vi "Edit(Channel).vi"(10 "TaskConfig":refnum<data-value>, 11 "Tag":string) -> ()   [LabVIEW 2025, in "DAQ_Module.lvlib" / "DAQ_Module.lvclass"]
uses:
  DAQ_Module.lvclass
  DAQ_Config.ctl
  DAQ_Task_Config.ctl
  DAQ_HW_Type.ctl
  DAQ_Task_Type.ctl
  DAQ_SampleRateConfig.ctl
  DAQ_AI_Task_Config.ctl
  DAQ_Linear_Task_Config.ctl
  DAQ_Angular_Task_Config.ctl
  <vilib>/addons/_JKI Toolkits/State Machine/_JKI_lib_State_Machine.llb/Select State(s)_err__jki_lib_state_machine.vi
  <vilib>/addons/_JKI Toolkits/State Machine/_JKI_lib_State_Machine.llb/Periodic Trigger__ogtk__JKI-SM__jki_lib_state_machine.vi
panel:
  in  "Cancel":bool
  in  "OK":bool
  in  "Tab Control":enum32{"AI", "Linear", "Angular", "AO"}(tab)
  in  "AI_Config":T1={"AI"={"MaxValue"=1.0, "MinValue"=0.0, "InputTerminalConfiguration"=-1}, "Scale"={"Offset"=0.0, "Gain"=1.0, "Unit"=""}, "Calibrate"={"K"=0.0, "B"=1.0}} {"AI"."InputTerminalConfiguration" items=["default"=-1, "RSE"=10083, "NRSE"=10078, "Differential"=10106, "Pseudodifferential"=12529]}
  in  "LinearConfig":T2={"decoding type"=10092, "units"=10219, "distance per pulse"=0.001, "initial position"=0.0, "z index enable"=FALSE, "z index value"=0.0, "z index phase"=10040, "CI_Encoder_A_InputTerm"="", "CI_Encoder_B_InputTerm"="", "CI_Encoder_Z_InputTerm"=""} {"units" items=["Meters"=10219, "Inches"=10379, "Ticks"=10304, "From Custom Scale"=10065]; "decoding type" items=["X1"=10090, "X2"=10091, "X4"=10092, "Two Pulse Counting"=10313]; "z index phase" items=["A High B High"=10040, "A High B Low"=10041, "A Low B High"=10042, "A Low B Low"=10043]}
  in  "AngularConfig":T3={"decoding type"=10092, "units"=10146, "pulses per revolution"=24, "initial angle"=0.0, "z index enable"=FALSE, "z index value"=0.0, "z index phase"=10040, "CI_Encoder_A_InputTerm"="", "CI_Encoder_B_InputTerm"="", "CI_Encoder_Z_InputTerm"=""} {"units" items=["Degrees"=10146, "Radians"=10273, "Ticks"=10304, "From Custom Scale"=10065]; "decoding type" items=["X1"=10090, "X2"=10091, "X4"=10092, "Two Pulse Counting"=10313]; "z index phase" items=["A High B High"=10040, "A High B Low"=10041, "A Low B High"=10042, "A Low B Low"=10043]}
  in  "Name":string
  in  "Channel":string
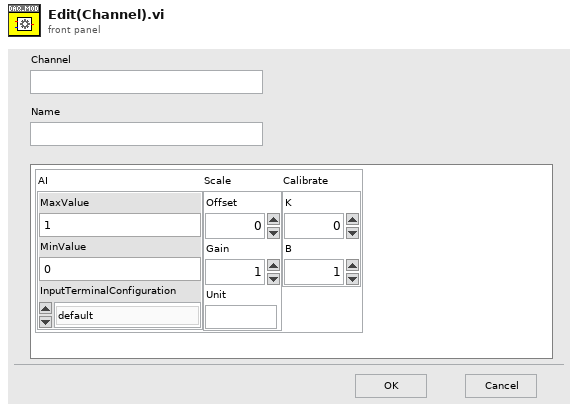
[diagram p1: front panel]
types:
  T1 = typedef "DAQ_Module.lvlib/DAQ_Module.lvclass/DAQ_AI_Task_Config.ctl" = cluster{"AI":cluster{"MaxValue":dbl, "MinValue":dbl, "InputTerminalConfiguration":i32}, "Scale":cluster{"Offset":dbl, "Gain":dbl, "Unit":string}, "Calibrate":cluster{"K":dbl, "B":dbl}}
  T2 = typedef "DAQ_Module.lvlib/DAQ_Module.lvclass/DAQ_Linear_Task_Config.ctl" = cluster{"decoding type":i32, "units":i32, "distance per pulse":dbl, "initial position":dbl, "z index enable":bool, "z index value":dbl, "z index phase":i32, "CI_Encoder_A_InputTerm":string, "CI_Encoder_B_InputTerm":string, "CI_Encoder_Z_InputTerm":string}
  T3 = typedef "DAQ_Module.lvlib/DAQ_Module.lvclass/DAQ_Angular_Task_Config.ctl" = cluster{"decoding type":i32, "units":i32, "pulses per revolution":u32, "initial angle":dbl, "z index enable":bool, "z index value":dbl, "z index phase":i32, "CI_Encoder_A_InputTerm":string, "CI_Encoder_B_InputTerm":string, "CI_Encoder_Z_InputTerm":string}
  T4 = enum32{"Invalid", "Standard", "Closed", "Hidden", "Minimized", "Maximized"}
  T5 = enum32{"invalid app kind", "Development System", "Run Time System", "Student Edition", "Embedded LabVIEW", "Evaluation", "Custom"}
  T6 = cluster{"Core":cluster{"Current VI Reference":refnum<vi>, "Close Panel on Exit?":bool}, "TaskConfig":refnum<data-value>, "Tag":string, "AI_Config":refnum<vi>, "AngularConfig":refnum<vi>, "LinearConfig":refnum<vi>, "Tab Control":refnum<vi>, "Channel":refnum<vi>, "Name":refnum<vi>}
  T7 = cluster{"Current VI Reference":refnum<vi>, "Close Panel on Exit?":bool}
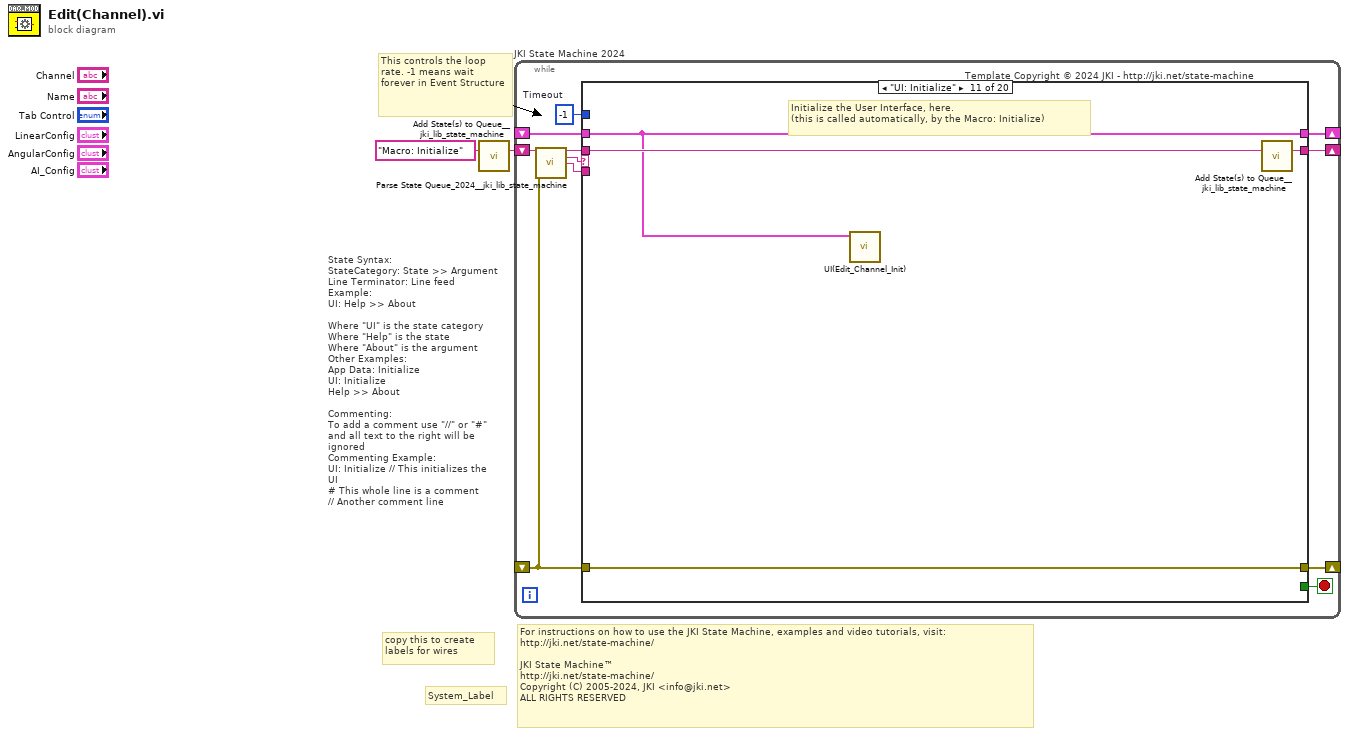
[diagram p0: block diagram]
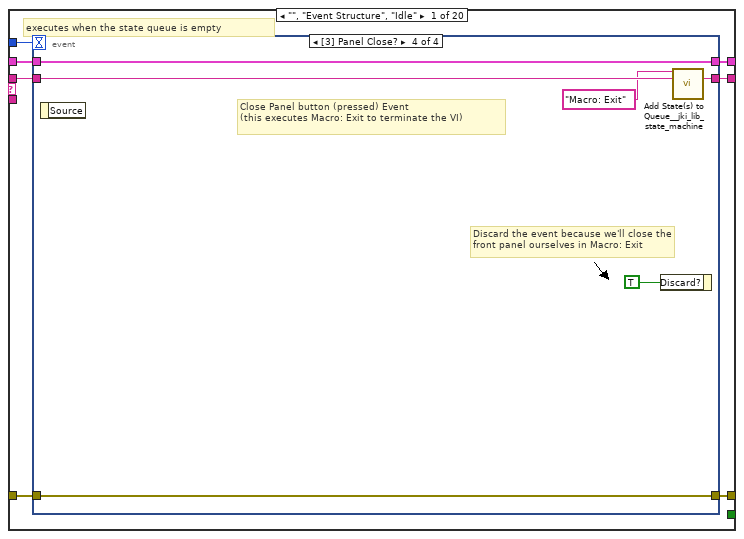
[diagram p2: hidden frame]
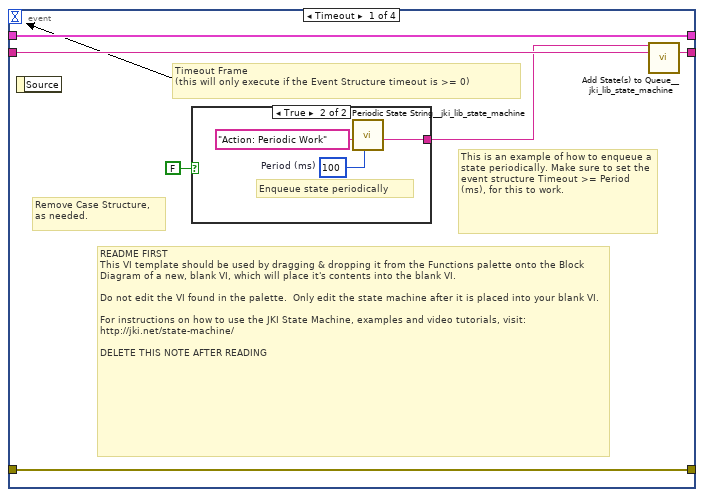
[diagram p3: hidden frame]
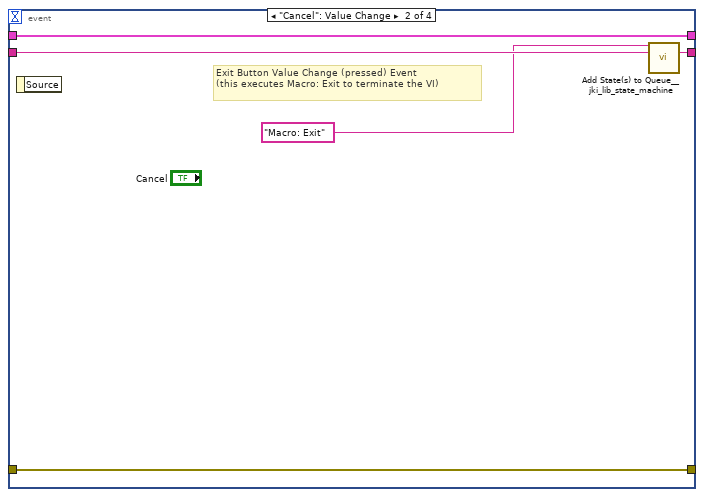
[diagram p5: hidden frame]
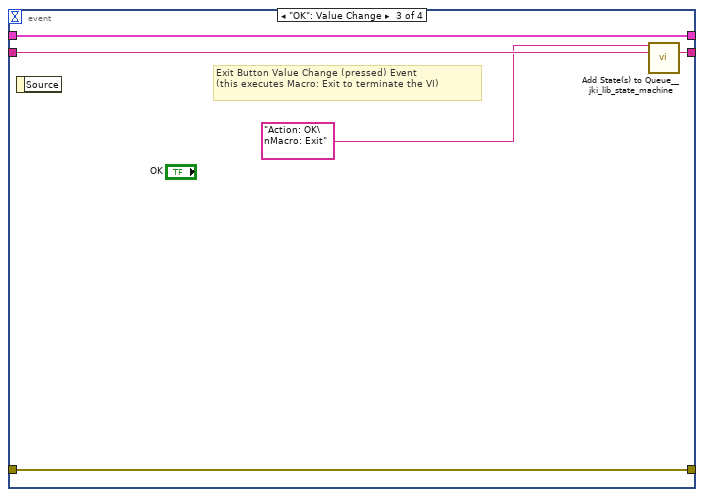
[diagram p6: hidden frame]
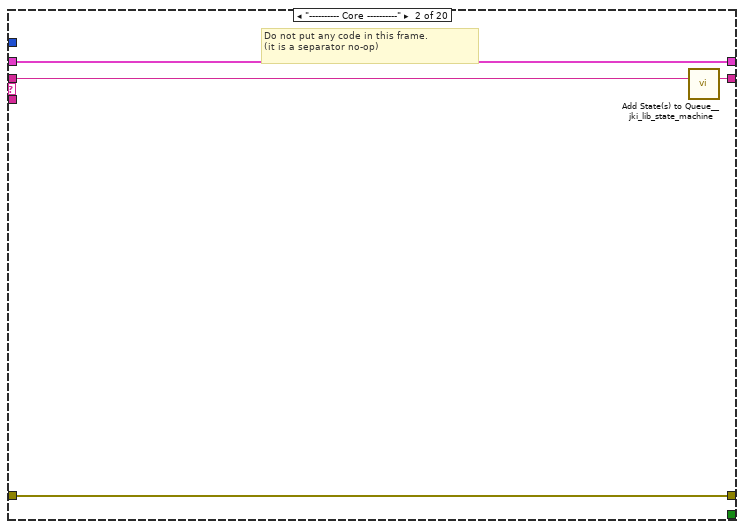
[diagram p7: hidden frame]
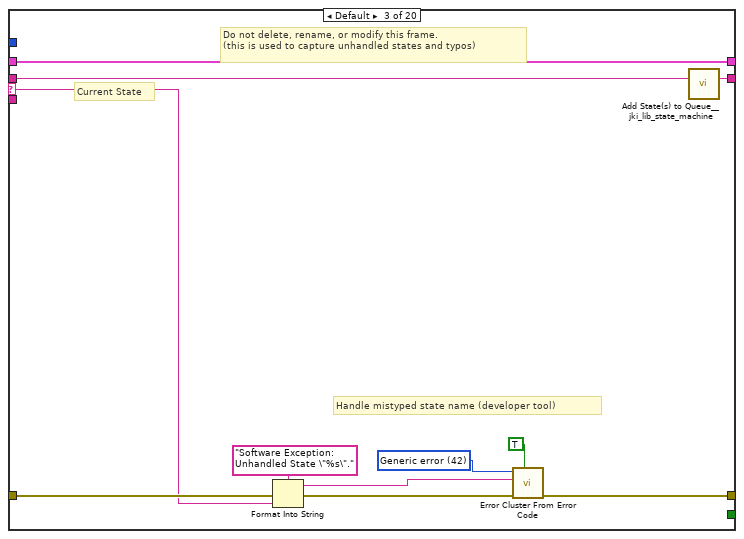
[diagram p8: hidden frame]
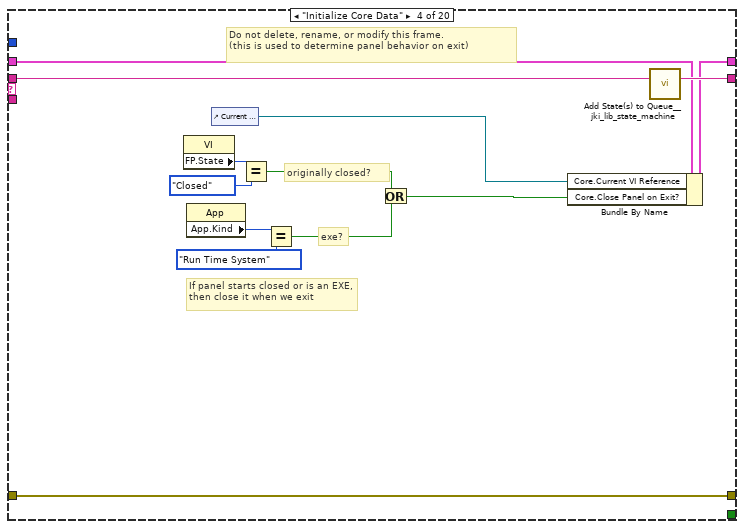
[diagram p9: hidden frame]
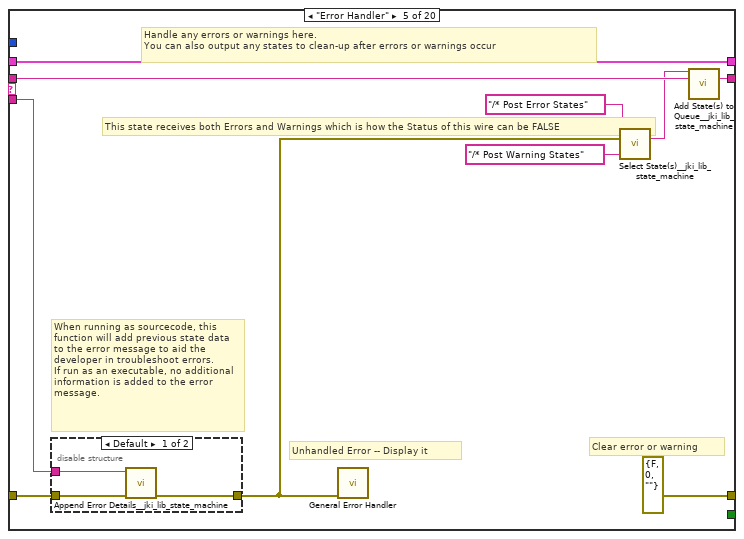
[diagram p10: hidden frame]
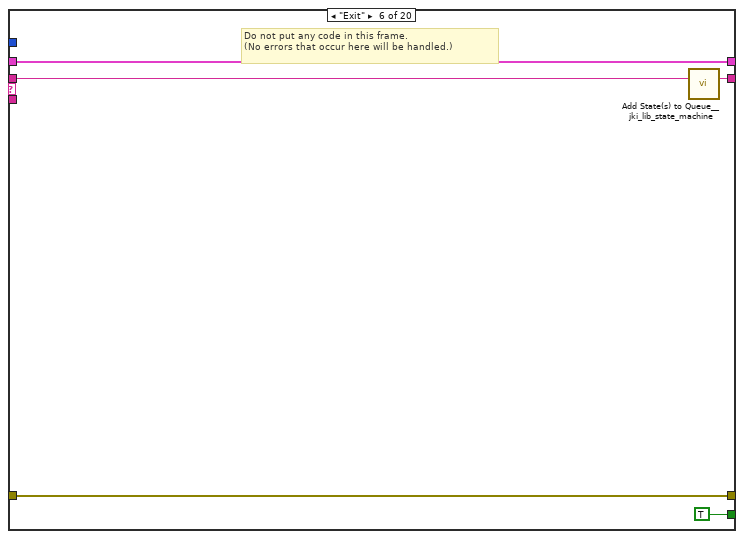
[diagram p12: hidden frame]
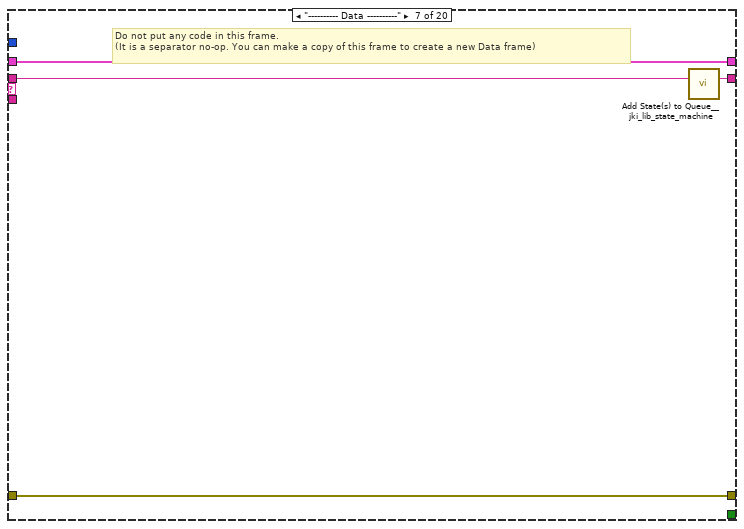
[diagram p13: hidden frame]
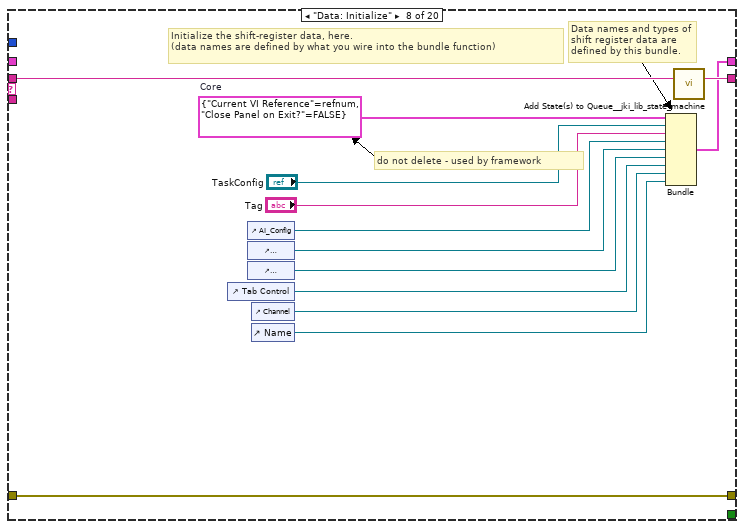
[diagram p14: hidden frame]
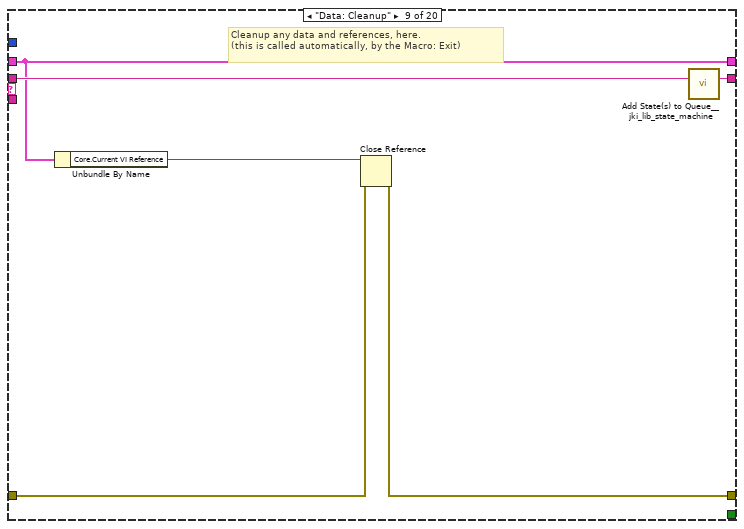
[diagram p15: hidden frame]
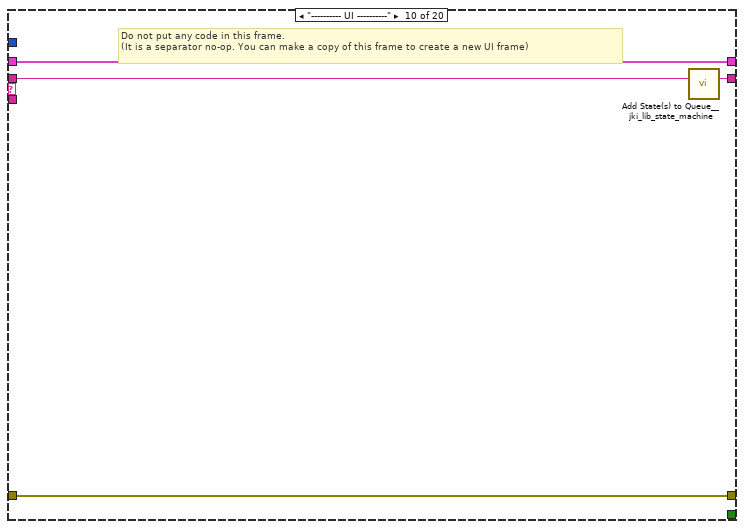
[diagram p16: hidden frame]
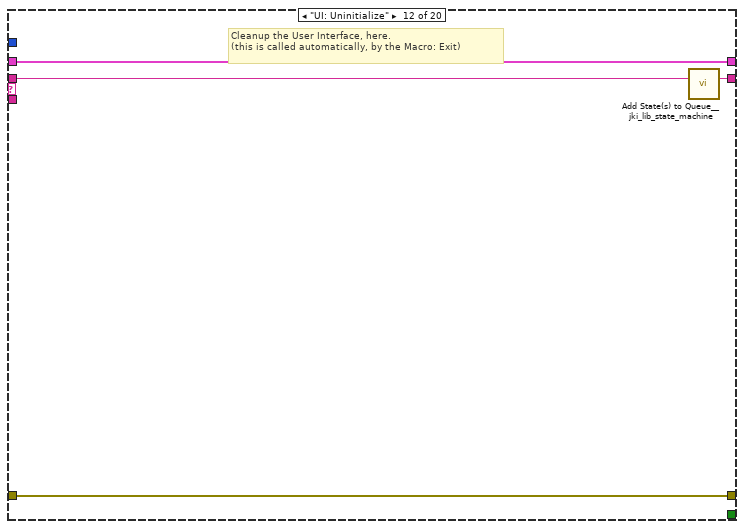
[diagram p17: hidden frame]
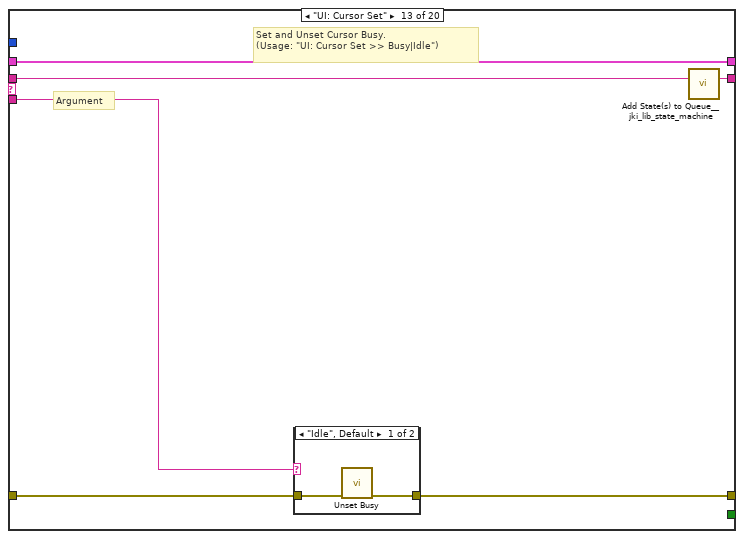
[diagram p18: hidden frame]
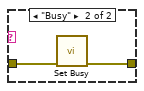
[diagram p19: hidden frame]
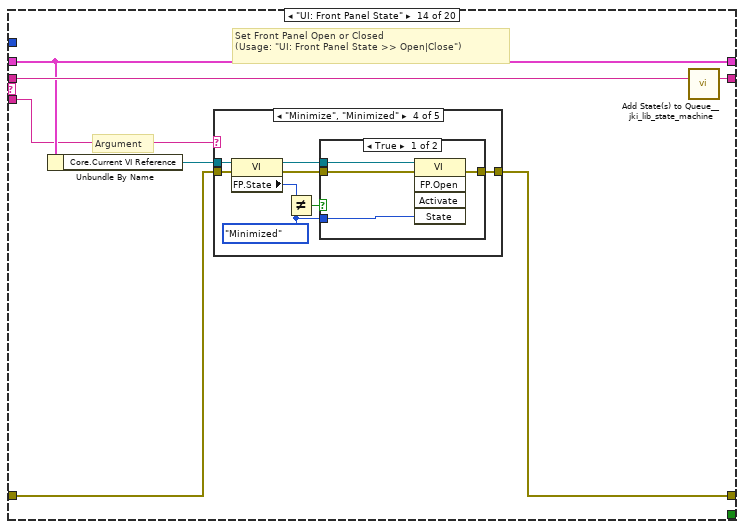
[diagram p20: hidden frame]
diagram:
  # "For instructions on how to use the JKI State Machine, examples and video tutorials, visit:\nhttp://jki.net/state-machine/\n\nJKI State Machine™\nhttp://jki.net/state-machine/\nCopyright (C) 2005-2024, JKI <info@jki.net>\nALL RIGHTS RESERVED"
  # "State Syntax:\nStateCategory: State >> Argument\nLine Terminator: Line feed\nExample:\nUI: Help >> About\n\nWhere \"UI\" is the state category\nWhere \"Help\" is the state\nWhere \"About\" is the argument\nOther Examples:\nApp Data: Initialize\nUI: Initialize\nHelp >> About\n\nCommenting:\nTo add a comment use \"//\" or \"#\" and all text to the right will be ignored\nCommenting Example:\nUI: Initialize // This initializes the UI\n# This whole line is a comment\n// Another comment line"
  # "copy this to create labels for wires"
  # "This controls the loop rate. -1 means wait forever in Event Structure"
  # "System_Label"
  n1 = call <vilib>:"Add State(s) to Queue__jki_lib_state_machine.vi"("State(s) in (\"\")"="Macro: Initialize") -> ("States Out"=w2:string)  [unwired: 14 in]
  n2 = while "JKI State Machine 2024" {
    shift-right: [w6] -> _
    shift-left: _ -> [w5]
    shift-right: [w9] -> _
    shift-left: _ -> [w3]
    shift-right: [w8] -> _
    shift-left: w2 -> [w10]
    stop <- w7 stop-if-true
    w4 = -1  # Timeout
    # "Template Copyright © 2024 JKI - http://jki.net/state-machine"
    n3 = call <vilib>:"Parse State Queue_2024__jki_lib_state_machine.vi"("State Queue"=w10, "Error In (no error)"=w3) -> ("Remaining States"=w12:string, "Current State"=w13:string, "Arguments"=w11:string)  [unwired: 11 in]
    n4 = case shown="\"UI: Initialize\"" w13 {
      selector: w13 -> [_ _ w50 _ _ _ _ _ _ _ _ _ _ _ _ _ _ _ _ _]
      tunnel: w12 -> [w20 w49 w54 w73 w83 w92 w96 w109 w115 w119 w123 w127 w133 w144 w213 w218 w227 w231 w235 w239]
      tunnel: w11 -> [_ _ _ _ w78 _ _ _ _ _ _ _ w128 w138 _ _ _ _ _ _]
      tunnel: w5 -> [w18 w46 w52 w66 w80 w90 w93 _ w110 w116 w120 w125 w131 w140 w210 w215 w225 w228 w232 w236]
      tunnel: [w17 w47 w56 w70 errorcluster {"status"=FALSE, "code"=0, "source"=""} ("error out") w89 w94 w106 w111 w117 w121 w124 w129 w141 w211 w216 w222 w229 w233 w237] -> w9
      tunnel: w3 -> [w14 w47 w55 w70 w79 w89 w94 w106 w112 w117 w121 w124 w130 w142 w211 w216 w222 w229 w233 w237]
      tunnel: [w19 w48 w53 w72 w82 w91 w95 w108 w114 w118 w122 w126 w132 w143 w212 w217 w226 w230 w234 w238] -> w8
      tunnel: [_ _ _ _ _ TRUE _ _ _ _ _ _ _ _ _ _ _ _ _ _] -> w7
      tunnel: [w16 w46 w52 w71 w80 w90 w93 w107 w110 w116 w120 w125 w131 w140 w210 w215 w225 w228 w232 w236] -> w6
      tunnel: w4 -> [w15 _ _ _ _ _ _ _ _ _ _ _ _ _ _ _ _ _ _ _]
      frame "", "Event Structure", "Idle" {
        # "executes when the state queue is empty"
        n5 = event shown="[3] Panel Close?" {
          selector: _ -> [_ _ _ _]
          dyn-events: _ -> [_ _ _ _]
          timeout: w15 -> [_ _ _ _]
          tunnel: w20 -> [w26 w34 w39 w45]
          tunnel: [w25 w33 w38 w44] -> w19
          tunnel: w18 -> [w23 w31 w36 w42]
          tunnel: [w24 w32 w37 w43] -> w17
          tunnel: w14 -> [w24 w32 w37 w43]
          tunnel: [w23 w31 w36 w42] -> w16
          event Timeout {
            # "Remove Case Structure, as needed."
            # "This is an example of how to enqueue a state periodically. Make sure to set the event structure Timeout >= Period (ms), for this to work."
            # "README FIRST\nThis VI template should be used by dragging & dropping it from the Functions palette onto the Block Diagram of a new, blank VI, which will place it's contents into the blank VI.\n\nDo not edit the VI found in the palette.  Only edit the state machine after it is placed into your blank VI.\n\nFor instructions on how to use the JKI State Machine, examples and video tutorials, visit:\nhttp://jki.net/state-machine/\n\nDELETE THIS NOTE AFTER READING"
            # "Timeout Frame\n(this will only execute if the Event Structure timeout is >= 0)"
            n6 = event-data() -> ()  [unwired: 1 in, 1 out]
            n7 = case shown="True" FALSE {
              tunnel: [_ w29] -> w22
              frame False {
              }
              frame True {
                w27 = u32 100  # Period (ms)
                # "Enqueue state periodically"
                n8 = call <vilib>:"Periodic State String__jki_lib_state_machine.vi"("Period (ms)"=w27, "State"="Action: Periodic Work") -> ("State Out"=w29:string)  [unwired: 9 in]
              }
            }
            n9 = call <vilib>:"Add State(s) to Queue__jki_lib_state_machine.vi"("State(s) in Front (\"\")"=w22, "State(s) in (\"\")"=w26) -> ("States Out"=w25:string)  [unwired: 13 in]
          }
          event "Cancel": Value Change {
            # "Exit Button Value Change (pressed) Event\n(this executes Macro: Exit to terminate the VI)"
            n10 = event-data() -> ()  [unwired: 1 in, 1 out]
            n11 = call <vilib>:"Add State(s) to Queue__jki_lib_state_machine.vi"("State(s) in Front (\"\")"="Macro: Exit", "State(s) in (\"\")"=w34) -> ("States Out"=w33:string)  [unwired: 13 in]
          }
          event "OK": Value Change {
            # "Exit Button Value Change (pressed) Event\n(this executes Macro: Exit to terminate the VI)"
            n12 = event-data() -> ()  [unwired: 1 in, 1 out]
            n13 = call <vilib>:"Add State(s) to Queue__jki_lib_state_machine.vi"("State(s) in Front (\"\")"="Action: OK\nMacro: Exit", "State(s) in (\"\")"=w39) -> ("States Out"=w38:string)  [unwired: 13 in]
          }
          event Panel Close? {
            # "Discard the event because we'll close the front panel ourselves in Macro: Exit"
            # "Close Panel button (pressed) Event\n(this executes Macro: Exit to terminate the VI)"
            n14 = event-data() -> ()  [unwired: 1 in, 1 out]
            n15 = event-data("Discard?"=TRUE) -> ()  [unwired: 1 in, 1 out]
            n16 = call <vilib>:"Add State(s) to Queue__jki_lib_state_machine.vi"("State(s) in Front (\"\")"="Macro: Exit", "State(s) in (\"\")"=w45) -> ("States Out"=w44:string)  [unwired: 13 in]
          }
        }
      }
      frame "---------- Core ----------" {
        # "Do not put any code in this frame.\n(it is a separator no-op)"
        n17 = call <vilib>:"Add State(s) to Queue__jki_lib_state_machine.vi"("State(s) in (\"\")"=w49) -> ("States Out"=w48:string)  [unwired: 14 in]
      }
      frame Default {
        w59 = 42 items=["No error", "Argument error", "Memory is full", "Out of zone", "End of file", "File already open", "Generic file I/O error", "File not found", "File permission error", "Disk is full", "Duplicate path", "Too many files open", "System feature not enabled", "Resource file not found", "Cannot add resource", "Resource not found", "Image not found", "Image memory error", "Pen does not exist", "Config type invalid", "Config token not found", "Config parse error", "Config memory error", "Bad external code format", "Bad external code offset", "External code not present", "Null window", "Destroy window error", "Null menu", "Print aborted", "Bad print record", "Print driver error", "Windows error during printing", "Memory error during printing", "Print dialog error", "Generic print error", "Invalid device refnum", "Device not found", "Device parameter error", "Device unit error", "Cannot open device", "Device call aborted", "Generic error", "Cancelled by user", "Object ID too low", "Object ID too high", "Object not in heap", "Unknown heap", "Unknown object (invalid DefProc)", "Unknown object (DefProc not in table)", "Message out of range", "Invalid (null) method", "Unknown message", "Manager call not supported", "Bad address", "Network operation in progress", "Network operation timed out", "Connection is busy", "Network attribute not supported", "Network error", "Address in use", "System out of memory", "Connection aborted", "Connection refused", "Not connected", "Already connected", "Connection closed", "Initialization error (interapplication manager)", "Bad occurrence", "Wait on unbound occurrence handler", "Occurrence queue overflow", "Datalog type conflict", "Unused", "Unrecognized type (interapplication manager)", "Memory corrupt", "Failed to make temporary DLL", "Old CIN version", "Drag socket not found", "Failed to load drop-object", "Failed to register OLE object", "Failed to release OLE object", "Format specifier type mismatch", "Unknown format specifier", "Too few format specifiers", "Too many format specifiers", "Scan failed", "Newer CIN version", "Error converting to variant", "Runtime menu error", "Password tampered", "Variant attribute not found", "Incompatible variant data type", "Event data is not available", "Event Store is not present", "Occurrence is not found", "Event Queue is not created", "Event info is not available", "Refnum passed is NULL", "Error retrieving Class GUID", "Error retrieving CoClass GUID", "Error retrieving TypeLib GUID.", "Bad built application magic bytes.", "Specific driver is different from the specific driver associated with the Logical Name.", "There is no session opened to the class driver.", "Max Error", "MAX - Error with config objects", "MAX - Error loading configuration", "MAX - Group not supported"]
        # "Current State"
        # "Do not delete, rename, or modify this frame.\n(this is used to capture unhandled states and typos)"
        # "Handle mistyped state name (developer tool)"
        n18 = Format Into String(format string="Software Exception: Unhandled State \"%s\"." ("message"), error in=w55, w50) -> (resulting string=w58:string, error out=w57:errorcluster)  [unwired: 1 in]
        n19 = call <vilib>:"Error Cluster From Error Code.vi"("show call chain? (False)"=TRUE, "error in (no error)"=w57, "error message (\"\")"=w58, "error code (0)"=w59) -> ("error out"=w56:errorcluster)  [unwired: 5 in]
        n20 = call <vilib>:"Add State(s) to Queue__jki_lib_state_machine.vi"("State(s) in (\"\")"=w54) -> ("States Out"=w53:string)  [unwired: 14 in]
      }
      frame "Initialize Core Data" {
        # "Do not delete, rename, or modify this frame.\n(this is used to determine panel behavior on exit)"
        # "originally closed?"
        # "exe?"
        # "If panel starts closed or is an EXE, then close it when we exit"
        n21 = property class="VI"() -> ("FP.State"=w63:T4)  [unwired: 2 in, 2 out]
        n22 = property class="App"() -> ("App.Kind"=w69:T5)  [unwired: 2 in, 2 out]
        n23 = control-ref of="Current VI Reference"() -> (w64:refnum<vi>)
        n24 = Equal?(x=w63, y=T4."Closed" ("Front Panel Window:State")) -> (x = y?=w61:bool)
        n25 = Equal?(x=w69, y=T5."Run Time System" ("Application:Kind")) -> (x = y?=w67:bool)
        n26 = Or(x=w61, y=w67) -> (x .or. y?=w65:bool)
        n27 = Bundle By Name(cluster=w66, "Core.Current VI Reference"=w64, "Core.Close Panel on Exit?"=w65) -> (w71:T6)
        n28 = call <vilib>:"Add State(s) to Queue__jki_lib_state_machine.vi"("State(s) in (\"\")"=w73) -> ("States Out"=w72:string)  [unwired: 14 in]
      }
      frame "Error Handler" {
        # "When running as sourcecode, this function will add previous state data to the error message to aid the developer in troubleshoot errors.\nIf run as an executable, no additional information is added to the error message."
        # "This state receives both Errors and Warnings which is how the Status of this wire can be FALSE"
        # "Unhandled Error -- Display it"
        # "Handle any errors or warnings here.\nYou can also output any states to clean-up after errors or warnings occur"
        # "Clear error or warning"
        n29 = disable-structure shown="Default" {
          disable-tunnel: w79 -> [w86 w87]
          disable-tunnel: w78 -> [w85 _]
          disable-tunnel: [w84 w87] -> w77
          frame condition #0 (active) {
            n30 = call <vilib>:"Append Error Details__jki_lib_state_machine.vi"("error in (no error)"=w86, "Previous State and Argument(s)"=w85) -> ("error out"=w84:errorcluster)  [unwired: 9 in]
          }
          frame condition #1 {
          }
        }
        n31 = call <vilib>:"General Error Handler.vi"("error in (no error)"=w77) -> ()  [unwired: 10 in, 5 out]
        n32 = call-poly <vilib>:"Select State(s)__jki_lib_state_machine.vi"("State(s) if True (\"\")"="/* Post Error States", "Select"=w77, "State(s) if False (\"\")"="/* Post Warning States") -> ("States Out"=w75:string)  [unwired: 12 in]
        n33 = call <vilib>:"Add State(s) to Queue__jki_lib_state_machine.vi"("State(s) in Front (\"\")"=w75, "State(s) in (\"\")"=w83) -> ("States Out"=w82:string)  [unwired: 13 in]
      }
      frame "Exit" {
        # "Do not put any code in this frame.\n(No errors that occur here will be handled.)"
        n34 = call <vilib>:"Add State(s) to Queue__jki_lib_state_machine.vi"("State(s) in (\"\")"=w92) -> ("States Out"=w91:string)  [unwired: 14 in]
      }
      frame "---------- Data ----------" {
        # "Do not put any code in this frame.\n(It is a separator no-op. You can make a copy of this frame to create a new Data frame)"
        n35 = call <vilib>:"Add State(s) to Queue__jki_lib_state_machine.vi"("State(s) in (\"\")"=w96) -> ("States Out"=w95:string)  [unwired: 14 in]
      }
      frame "Data: Initialize" {
        w105 = T7 {"Current VI Reference"=refnum, "Close Panel on Exit?"=FALSE}  # Core
        # "do not delete - used by framework"
        # "Data names and types of shift register data are defined by this bundle."
        # "Initialize the shift-register data, here.\n(data names are defined by what you wire into the bundle function)"
        n36 = control-ref of="Tab Control"() -> (w99:refnum<vi>)
        n37 = control-ref of="AI_Config"() -> (w102:refnum<vi>)
        n38 = control-ref of="AngularConfig"() -> (w101:refnum<vi>)
        n39 = control-ref of="LinearConfig"() -> (w100:refnum<vi>)
        n40 = control-ref of="Channel"() -> (w98:refnum<vi>)
        n41 = control-ref of="Name"() -> (w97:refnum<vi>)
        n42 = Bundle("Core"=w105, "TaskConfig"="TaskConfig", "Tag"="Tag", "AI_Config"=w102, "AngularConfig"=w101, "LinearConfig"=w100, "Tab Control"=w99, "Channel"=w98, "Name"=w97) -> (w107:T6)  [unwired: 1 in]
        n43 = call <vilib>:"Add State(s) to Queue__jki_lib_state_machine.vi"("State(s) in (\"\")"=w109) -> ("States Out"=w108:string)  [unwired: 14 in]
      }
      frame "Data: Cleanup" {
        # "Cleanup any data and references, here.\n(this is called automatically, by the Macro: Exit)"
        n44 = Unbundle By Name(w110) -> ("Core.Current VI Reference"=w113:refnum<vi>)
        n45 = Close Reference(reference=w113, error in (no error)=w112) -> (error out=w111:errorcluster)
        n46 = call <vilib>:"Add State(s) to Queue__jki_lib_state_machine.vi"("State(s) in (\"\")"=w115) -> ("States Out"=w114:string)  [unwired: 14 in]
      }
      frame "---------- UI ----------" {
        # "Do not put any code in this frame.\n(It is a separator no-op. You can make a copy of this frame to create a new UI frame)"
        n47 = call <vilib>:"Add State(s) to Queue__jki_lib_state_machine.vi"("State(s) in (\"\")"=w119) -> ("States Out"=w118:string)  [unwired: 14 in]
      }
      frame "UI: Initialize" {
        # "Initialize the User Interface, here.\n(this is called automatically, by the Macro: Initialize)"
        n48 = call "UI(Edit_Channel_Init).vi"("Cluster"=w120) -> ()  [unwired: 11 in]
        n49 = call <vilib>:"Add State(s) to Queue__jki_lib_state_machine.vi"("State(s) in (\"\")"=w123) -> ("States Out"=w122:string)  [unwired: 14 in]
      }
      frame "UI: Uninitialize" {
        # "Cleanup the User Interface, here.\n(this is called automatically, by the Macro: Exit)"
        n50 = call <vilib>:"Add State(s) to Queue__jki_lib_state_machine.vi"("State(s) in (\"\")"=w127) -> ("States Out"=w126:string)  [unwired: 14 in]
      }
      frame "UI: Cursor Set" {
        # "Argument"
        # "Set and Unset Cursor Busy.\n(Usage: \"UI: Cursor Set >> Busy|Idle\")"
        n51 = case shown="\"Idle\", Default" w128 {
          tunnel: w130 -> [w135 w137]
          tunnel: [w134 w136] -> w129
          frame "Idle", Default {
            n52 = call <vilib>:"Unset Busy.vi"("error in (no error)"=w135) -> ("error out"=w134:errorcluster)  [unwired: 10 in]
          }
          frame "Busy" {
            n53 = call <vilib>:"Set Busy.vi"("error in (no error)"=w137) -> ("error out"=w136:errorcluster)  [unwired: 9 in, 1 out]
          }
        }
        n54 = call <vilib>:"Add State(s) to Queue__jki_lib_state_machine.vi"("State(s) in (\"\")"=w133) -> ("States Out"=w132:string)  [unwired: 14 in]
      }
      frame "UI: Front Panel State" {
        # "Argument"
        # "Set Front Panel Open or Closed\n(Usage: \"UI: Front Panel State >> Open|Close\")"
        n55 = Unbundle By Name(w140) -> ("Core.Current VI Reference"=w139:refnum<vi>)
        n56 = case shown="\"Minimize\", \"Minimized\"" w138 {
          tunnel: w142 -> [w150 w165 w176 w189 w202]
          tunnel: [w152 w166 w178 w191 w204] -> w141
          tunnel: w139 -> [w151 w163 w177 w190 w203]
          frame "Open", "Standard", Default {
            w145 = T4."Standard" ("State")
            n57 = property class="VI"(reference=w151, error in=w150) -> (reference out=w148:refnum<vi>, error out=w149:errorcluster, "FP.State"=w147:T4)
            n58 = Not Equal?(x=w147, y=w145) -> (x != y?=w146:bool)
            n59 = case shown="True" w146 {
              tunnel: [w156 w158] -> w152
              tunnel: w149 -> [w155 w158]
              tunnel: w148 -> [w154 _]
              tunnel: w145 -> [w153 _]
              frame True {
                n60 = invoke class="VI" method="FP.Open"(reference=w154, error in=w155, "Activate"=TRUE, "State"=w153) -> (error out=w156:errorcluster)  [unwired: 1 in, 4 out]
              }
              frame False {
              }
            }
          }
          frame "Close", "Closed" {
            n61 = property class="VI"(reference=w163, error in=w165) -> (reference out=w162:refnum<vi>, error out=w164:errorcluster, "FP.State"=w160:T4)
            n62 = Not Equal?(x=w160, y=T4."Closed" ("Front Panel Window:State")) -> (x != y?=w159:bool)
            n63 = case shown="True" w159 {
              tunnel: [w167 w170] -> w166
              tunnel: w164 -> [w167 w169]
              tunnel: w162 -> [_ w168]
              frame False {
              }
              frame True {
                n64 = invoke class="VI" method="FP.Close"(reference=w168, error in=w169) -> (error out=w170:errorcluster)  [unwired: 1 in, 2 out]
              }
            }
          }
          frame "Hidden", "Hide" {
            w171 = T4."Hidden" ("State")
            n65 = property class="VI"(reference=w177, error in=w176) -> (reference out=w174:refnum<vi>, error out=w175:errorcluster, "FP.State"=w173:T4)
            n66 = Not Equal?(x=w173, y=w171) -> (x != y?=w172:bool)
            n67 = case shown="True" w172 {
              tunnel: [w182 w183] -> w178
              tunnel: w175 -> [w181 w183]
              tunnel: w174 -> [w180 _]
              tunnel: w171 -> [w179 _]
              frame True {
                n68 = invoke class="VI" method="FP.Open"(reference=w180, error in=w181, "State"=w179) -> (error out=w182:errorcluster)  [unwired: 2 in, 4 out]
              }
              frame False {
              }
            }
          }
          frame "Minimize", "Minimized" {
            w184 = T4."Minimized" ("State")
            n69 = property class="VI"(reference=w190, error in=w189) -> (reference out=w187:refnum<vi>, error out=w188:errorcluster, "FP.State"=w186:T4)
            n70 = Not Equal?(x=w186, y=w184) -> (x != y?=w185:bool)
            n71 = case shown="True" w185 {
              tunnel: [w195 w196] -> w191
              tunnel: w188 -> [w194 w196]
              tunnel: w187 -> [w193 _]
              tunnel: w184 -> [w192 _]
              frame True {
                n72 = invoke class="VI" method="FP.Open"(reference=w193, error in=w194, "State"=w192) -> (error out=w195:errorcluster)  [unwired: 2 in, 4 out]
              }
              frame False {
              }
            }
          }
          frame "Maximize", "Maximized" {
            w197 = T4."Maximized" ("State")
            n73 = property class="VI"(reference=w203, error in=w202) -> (reference out=w200:refnum<vi>, error out=w201:errorcluster, "FP.State"=w199:T4)
            n74 = Not Equal?(x=w199, y=w197) -> (x != y?=w198:bool)
            n75 = case shown="True" w198 {
              tunnel: [w208 w209] -> w204
              tunnel: w201 -> [w207 w209]
              tunnel: w200 -> [w206 _]
              tunnel: w197 -> [w205 _]
              frame True {
                n76 = invoke class="VI" method="FP.Open"(reference=w206, error in=w207, "State"=w205) -> (error out=w208:errorcluster)  [unwired: 2 in, 4 out]
              }
              frame False {
              }
            }
          }
        }
        n77 = call <vilib>:"Add State(s) to Queue__jki_lib_state_machine.vi"("State(s) in (\"\")"=w144) -> ("States Out"=w143:string)  [unwired: 14 in]
      }
      frame "---------- Macro ----------" {
        # "Do not put any code in this frame.\n(It is a separator no-op. You can make a copy of this frame to create a new Macro frame)"
        n78 = call <vilib>:"Add State(s) to Queue__jki_lib_state_machine.vi"("State(s) in (\"\")"=w213) -> ("States Out"=w212:string)  [unwired: 14 in]
      }
      frame "Macro: Initialize" {
        w214 = "Data: Initialize\nInitialize Core Data\nUI: Initialize\nUI: Front Panel State >> Open"  # Data: Initialize Initialize Core Data UI: Initialize UI: Front Panel State >> Open
        # "Initialization Macro\n(This is called once, when the VI starts)"
        n79 = call <vilib>:"Add State(s) to Queue__jki_lib_state_machine.vi"("State(s) in Front (\"\")"=w214, "State(s) in (\"\")"=w218) -> ("States Out"=w217:string)  [unwired: 13 in]
      }
      frame "Macro: Exit" {
        # "Exit Macro\n(This is called once, when the VI exits)"
        n80 = Unbundle By Name(w225) -> ("Core.Close Panel on Exit?"=w220:bool)
        n81 = call <vilib>:"Conditional State String__jki_lib_state_machine.vi"("Do State(s)?"=w220, "State"="UI: Front Panel State >> Close") -> ("State Out"=w219:string)  [unwired: 7 in]
        n82 = call <vilib>:"Add State(s) to Queue__jki_lib_state_machine.vi"("State(s) in (\"\")"=w219, "State(s) at Back (\"\")"="UI: Uninitialize\nData: Cleanup\nExit") -> ("States Out"=w223:string)  [unwired: 13 in]
        n83 = call <vilib>:"Add State(s) to Queue__jki_lib_state_machine.vi"("State(s) in Front (\"\")"=w223, "State(s) in (\"\")"=w227) -> ("States Out"=w226:string)  [unwired: 13 in]
      }
      frame "---------- Action ----------" {
        # "Template Separator\n(You can make a copy of, or modify, this frame)"
        n84 = call <vilib>:"Add State(s) to Queue__jki_lib_state_machine.vi"("State(s) in (\"\")"=w231) -> ("States Out"=w230:string)  [unwired: 14 in]
      }
      frame "Action: OK" {
        # "Your code here.\n(You can make a copy of, or modify, this frame)"
        n85 = call "GetValue(Channel).vi"("Cluster"=w232) -> ()  [unwired: 11 in]
        n86 = call <vilib>:"Add State(s) to Queue__jki_lib_state_machine.vi"("State(s) in (\"\")"=w235) -> ("States Out"=w234:string)  [unwired: 14 in]
      }
      frame "Action: Channel" {
        # "Your code here.\n(You can make a copy of, or modify, this frame)"
        n87 = call <vilib>:"Add State(s) to Queue__jki_lib_state_machine.vi"("State(s) in (\"\")"=w239) -> ("States Out"=w238:string)  [unwired: 14 in]
      }
    }
  }
